vi "SlaveAccelerometerSample3.vi"   [LabVIEW 2018]
uses:
  DataTypes/AccelerometerRecord3.ctl
  <vilib>/rvi/Emulation/niFpgaGetClockAttributes.vi
  <vilib>/rvi/Emulation/niFpgaSctlEmulationGetInTimedLoop.vi
  <vilib>/rvi/Emulation/niFpgaEmulationReportErrorSimple.vi
  <vilib>/rvi/eio/common/nirviEmuTemplateMethod_errors.vi
  <vilib>/rvi/Emulation/niFpgaEmulationIsFPGAContextNoSignature.vi
  <vilib>/rvi/DataTransferAndStorage/Container/Common/niFpgaContainerGetUniqueNameForEmu.vi
  <vilib>/rvi/Memory/Memory_Emulation/niFpgaMemoryEmulationCacheClearOnFirstRun.vi
  <vilib>/rvi/Memory/Memory_Emulation/nirvimemoryEmulationManagerCache_MakeExclusive.vi
  <vilib>/rvi/Memory/Memory_Emulation/niFpgaMemoryEmulationValidateCache.vi
  <vilib>/rvi/Memory/Memory_Emulation/nirvimemoryEmulationManagerCache_InsertValue.vi
  <vilib>/Utility/error.llb/Clear Errors.vi
  <vilib>/rvi/Memory/Memory_Emulation/nirvimemoryEmulationManagerCache_ReleaseExclusive.vi
  <vilib>/rvi/Memory/Memory_Emulation/nirvimemoryEmulationManagerCache_GetValue.vi
  <vilib>/rvi/Memory/Memory_Emulation/nirvimemoryEmulationManagerCache_SetValue.vi
  <vilib>/rvi/Emulation/niFpgaProcessEmulError.vi
  <vilib>/rvi/errors/niFpgaSetErrorForExecOnDevCompSimple.vi
  <vilib>/rvi/eio/common/nirviEmuReportErrorAndStop.vi
  <vilib>/rvi/FIFO/Fifo_Resource/nirvififoEmulationSetSize.vi
  <vilib>/rvi/FIFO/Fifo_Resource/nirviFifoEmulationQueueMgr.vi
  <instcachedir>/0/nirviFifoEmulationQueueMgr_E5CAEC123FF24DC58D834DCA3CDAA9B5.lvgen/nirviFifoEmulationQueueMgr_E5CAEC123FF24DC58D834DCA3CDAA9B5_033.vi
  <vilib>/rvi/FIFO/Fifo_Resource/nirvififoEmulationDetermineInputValidOut.vi
  <vilib>/rvi/FIFO/Fifo_Resource/nirvififoEmulationCreateLock.vi
  <vilib>/rvi/FIFO/Fifo_Resource/nirvififoEmulationObtainLock.vi
  <vilib>/rvi/FIFO/Fifo_Resource/nirvififoEmulationReleaseLock.vi
  <vilib>/rvi/occurrence/nirviWaitOnOccurrenceBase.vi
  <vilib>/rvi/errors/nirviReportUnexpectedCaseInternalError.vi
  <vilib>/rvi/errors/nirviReportUnexpectedCaseInternalError (U32).vi
  <vilib>/rvi/Emulation/niFpgaCriticalErrorInLSC.vi
  <vilib>/eio/EIOMethodNode/EIOMethodNode.xnode
  <vilib>/rvi/DataTransferAndStorage/Container/XNode/niFpgaContainer.xnode
  <vilib>/rvi/DataTransferAndStorage/Register/Emulation/niFpgaRegisterEmulation.vi
  <vilib>/eio/EIONode/EIONode.xnode
  <vilib>/rvi/FIFO/Fifo_Resource/nirvififoEmulationWrite.vi
types:
  T1 = typedef "AccelerometerRecord3.ctl" = cluster{"Timestamp":u64, "Accelerometers":sgl[]}
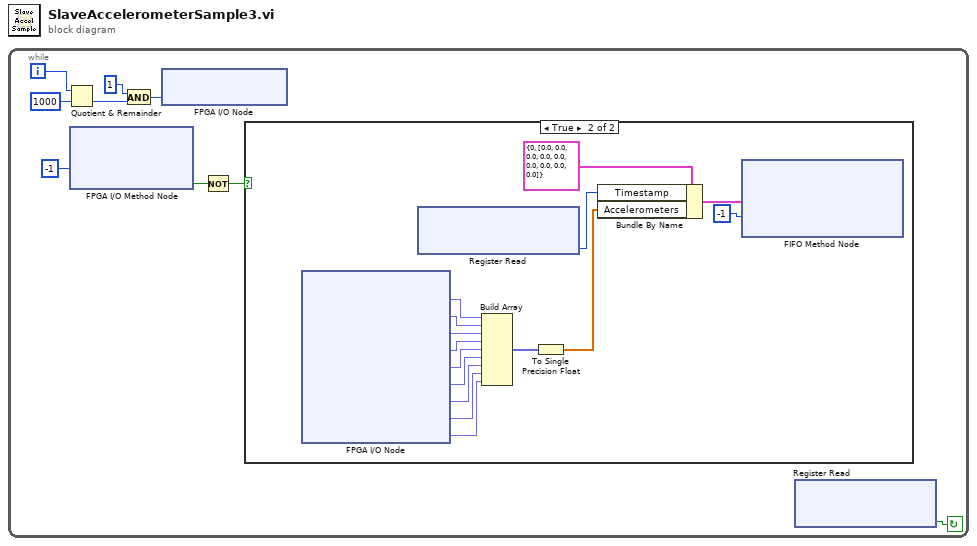
[diagram p0: block diagram]
diagram:
  n1 = while {
    i -> [w1]
    stop <- w2 continue-if-true
    n2 = Quotient & Remainder(x=w1, y=i16 1000) -> (floor(x/y)=w5:i32)  [unwired: 1 out]
    n3 = xnode "FPGA I/O Method Node"("Timeout"=-1) -> ("Timed Out"=w8:bool)  [unwired: 1 in, 1 out]
    n4 = And(x=1 ("y"), y=w5) -> (x .and. y?=w3:i32)
    n5 = xnode "FPGA I/O Node"("USER FPGA LED"=w3) -> ()  [unwired: 1 in, 1 out]
    n6 = Not(x=w8) -> (.not. x?=w7:bool)
    n7 = case shown="True" w7 {
      frame False {
      }
      frame True {
        n8 = xnode "FPGA I/O Node"() -> ("Accelerometer1/AI0"=w23:fxp<+/-,24,4>, "Accelerometer1/AI1"=w22:fxp<+/-,24,4>, "Accelerometer1/AI2"=w21:fxp<+/-,24,4>, "Accelerometer2/AI0"=w20:fxp<+/-,24,4>, "Accelerometer2/AI1"=w19:fxp<+/-,24,4>, "Accelerometer2/AI2"=w18:fxp<+/-,24,4>, "Accelerometer3/AI0"=w17:fxp<+/-,24,4>, "Accelerometer3/AI1"=w16:fxp<+/-,24,4>, "Accelerometer3/AI2"=w15:fxp<+/-,24,4>)  [unwired: 9 in, 9 out]
        n9 = xnode ("Register Read")() -> ("Data"=w12:u64)  [unwired: 1 in, 1 out]
        n10 = Build Array(w23, w22, w21, w20, w19, w18, w17, w16, w15) -> (w24:fxp<+/-,24,4>[])
        n11 = To Single Precision Float(number=w24) -> (single precision float=w13:sgl[])
        n12 = Bundle By Name(cluster=T1 {"Timestamp"=0, "Accelerometers"=[0.0, 0.0, 0.0, 0.0, 0.0, 0.0, 0.0, 0.0, 0.0]} ("AccelerometerSample3"), "Timestamp"=w12, "Accelerometers"=w13) -> (w10:T1)
        n13 = xnode ("FIFO Method Node")("Element"=w10, "Timeout"=-1) -> ()  [unwired: 1 in, 2 out]
      }
    }
    n14 = xnode ("Register Read")() -> ("Data"=w2:bool)  [unwired: 1 in, 1 out]
  }
